vi "VOC.vi"(0 "input VOC ports":u8[](array[numeric]), 1 "voc states array":cluster{u32, u8}[](array[cluster]), 5 "output VOC ports":u8[](array[numeric]), 9 "Input VOC msg Array":cluster{i32, "Value":string, i32}[](array[cluster]), 11 "output VOC msg array":cluster{i32, "Value":string, i32}[](array[cluster]), 12 "VOC output msg CASHE":cluster{i32, "Value":string, i32}[](array[cluster])) -> (3 "Filled voc states array":cluster{u32, u8}[](array[cluster]), 4 "Modified input VOC ports":u8[](array[numeric]), 6 "Modified output VOC ports":u8[](array[numeric]), 8 "Clear Input VOC msg Array":cluster{i32, "Value":string, i32}[](array[cluster]), 10 "clear output VOC array":cluster{i32, "Value":string, i32}[](array[cluster]), 14 "Curr step output MSG counter":i32, 15 "Filled VOC output msg CASHE":cluster{i32, "Value":string, i32}[](array[cluster]))   [LabVIEW 2009]
uses:
  Old BSVT Complex/lib/voc.dll
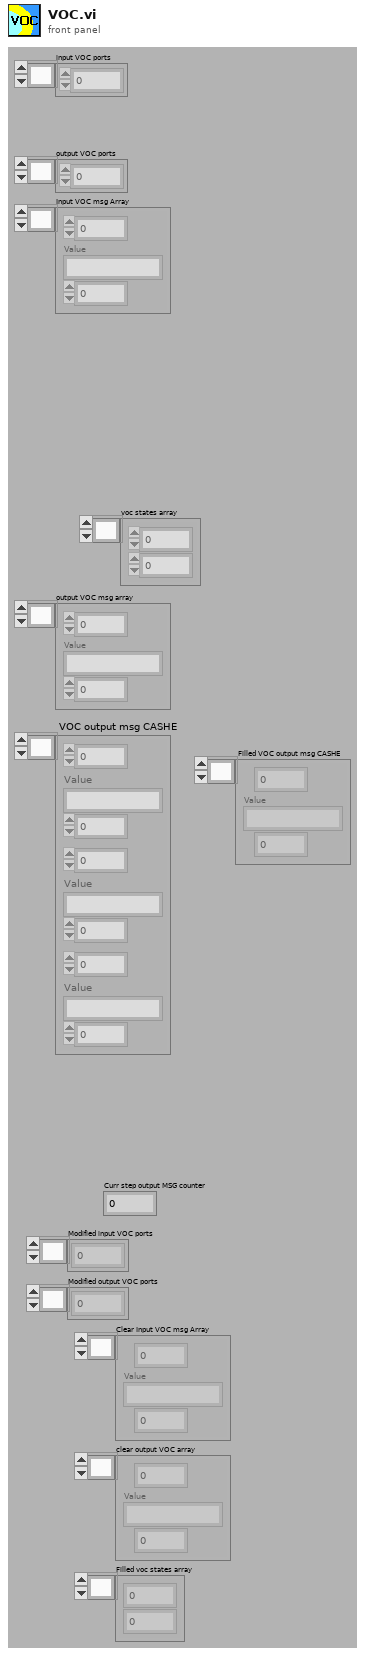
[diagram p1: front panel]
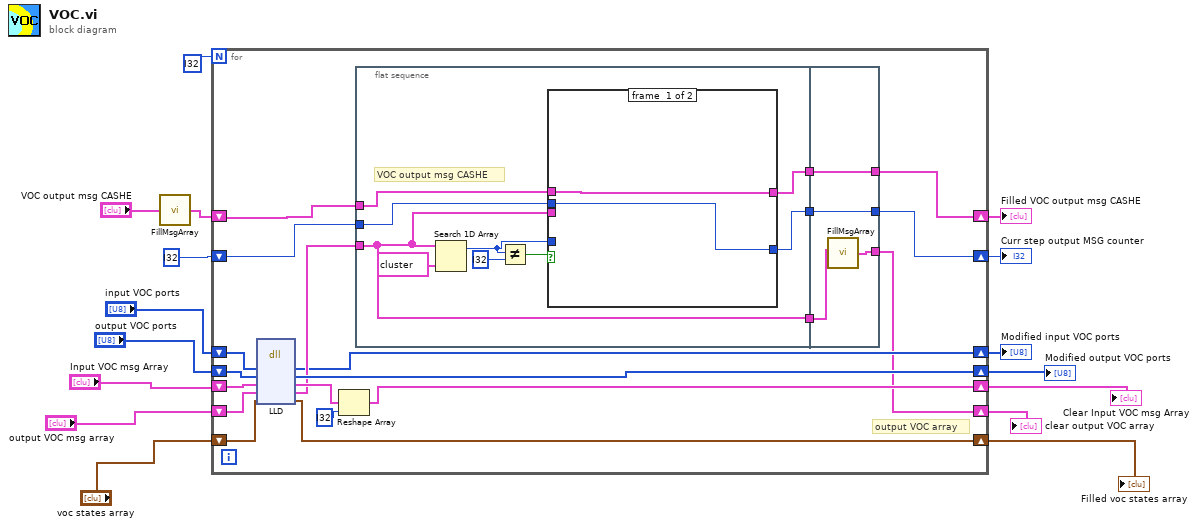
[diagram p0: block diagram]
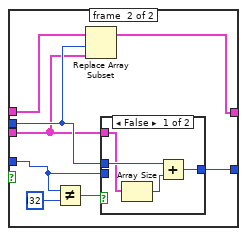
[diagram p2: hidden frame]
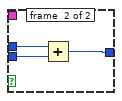
[diagram p3: hidden frame]
diagram:
  n1 = call "FillMsgArray.vi"("input array"="VOC output msg CASHE") -> ("output array"=w14:cluster{i32, "Value":string, i32}[])
  n2 = for {
    N: i32 ? -> [_]
    shift-right: [w23] -> w5
    shift-left: "input VOC ports" -> [w32]
    shift-right: [w36] -> w4
    shift-left: "output VOC ports" -> [w31]
    shift-right: [w33] -> w1
    shift-left: "voc states array" -> [w34]
    shift-right: [w27] -> w3
    shift-left: "Input VOC msg Array" -> [w35]
    shift-right: [w19] -> w2
    shift-left: "output VOC msg array" -> [w30]
    shift-right: [w17] -> w7
    shift-left: w14 -> [w26]
    shift-right: [w18] -> w6
    shift-left: i32 ? -> [w25]
    # "output VOC array"
    n3 = dll-call lib="D:/Liakh Tanya/Dissertation/Complex/Old debug progs/Old BSVT Complex/lib/voc.dll" fn="LLD" label="VOC"("input"=w32, "output"=w31, "Input VOC msg Array"=w35, "output VOC msg array"=w30, "voc states array"=w34) -> ("input"=w23:i8[], "output"=w36:i8[], "Input VOC msg Array"=w28:cluster{i32, "Value":string, i32}[], "output VOC msg array"=w24:cluster{i32, "Value":string, i32}[], "voc states array"=w33:cluster{u32, u8}[])  [unwired: 4 in, 2 out]
    n4 = Reshape Array(w28, i32 ? ("dimension size")) -> (w27:cluster{i32, "Value":string, i32}[])
    n5 = flat-sequence {
      tunnel: w26 -> [w43]
      tunnel: w25 -> [w42]
      tunnel: w24 -> [w41]
      tunnel: [w37] -> w22
      tunnel: [w39] -> w21
      tunnel: [w41] -> w20
      tunnel: [w65] -> w17
      tunnel: [w66] -> w18
      tunnel: w22 -> [w66]
      tunnel: w21 -> [w65]
      tunnel: w20 -> [w64]
      tunnel: [w63] -> w19
      frame #0 {
        # "VOC output msg CASHE"
        n6 = Search 1D Array(1D array=w41, element=cluster{i32, "Value":string, i32} ?) -> (index of element=w38:i32)  [unwired: 1 in]
        n7 = Not Equal?(x=w38, y=i32 ?) -> (x != y?=w40:bool)
        n8 = case shown="True" w40 {
          tunnel: w43 -> [w47 w55]
          tunnel: w42 -> [w46 w53]
          tunnel: w41 -> [_ w48]
          tunnel: [w47 w54] -> w39
          tunnel: w38 -> [_ w50]
          tunnel: [w46 w52] -> w37
          frame #0 {
          }
          frame #1 {
            n9 = Not Equal?(x=w50, y=i32 ?) -> (x != y?=w49:bool)
            n10 = Replace Array Subset(array=w55, new element=w48, index=w53) -> (w54:cluster{i32, "Value":string, i32}[])
            n11 = case shown="False" w49 {
              tunnel: w53 -> [w59 w62]
              tunnel: w50 -> [_ w61]
              tunnel: [w58 w60] -> w52
              tunnel: w48 -> [w57 _]
              frame #0 {
                n12 = Array Size(array=w57) -> (size(s)=w56:i32)
                n13 = Add(x=w59, y=w56) -> (x+y=w58:i32)
              }
              frame #1 {
                n14 = Add(x=w62, y=w61) -> (x+y=w60:i32)
              }
            }
          }
        }
      }
      frame #1 {
        n15 = call "FillMsgArray.vi"("input array"=w64) -> ("output array"=w63:cluster{i32, "Value":string, i32}[])
      }
    }
  }
  "Filled VOC output msg CASHE" <- w7
  "Curr step output MSG counter" <- w6
  "Modified input VOC ports" <- w5
  "Modified output VOC ports" <- w4
  "Clear Input VOC msg Array" <- w3
  "clear output VOC array" <- w2
  "Filled voc states array" <- w1
